vi "CheckIfStartModuleScriptExistsinINIFile.vi"(8 "error in":errorcluster, 11 "OrigTestTreeTags":string[](array[string])) -> (0 "error out":errorcluster, 1 "Found?":bool, 2 "INIs with Start Module script":T1, 3 "OrigTestTreeTags out":string[](array[string]))   [LabVIEW 2018]
uses:
  TestConfiguration.ctl
  <vilib>/Utility/config.llb/NI_LVConfig.lvlib
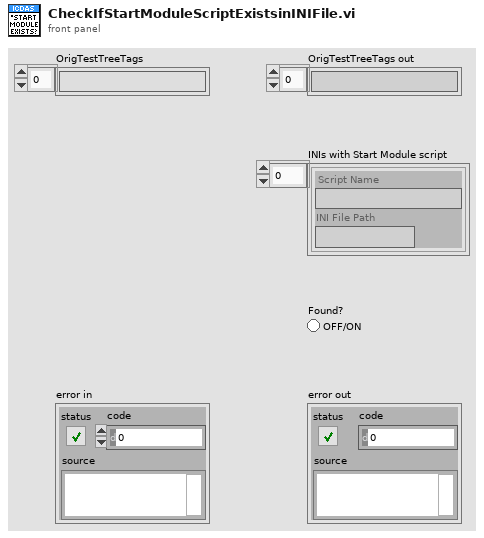
[diagram p1: front panel]
types:
  T1 = typedef "TestConfiguration.ctl" = cluster{"Script Name":string, "INI File Path":string}[]
  T2 = cluster{"Script Name":string, "INI File Path":string}
  T3 = typedef "Plugin Tree Tag.ctl" = cluster{"ItemType":T4, "Name":string, "Path":path, "Script":string[]}
  T4 = typedef "Plugins Tree Item Type.ctl" = enum16{"Plugin", "Instrument", "INI File", "INI Script"}
  T5 = typedef "NI_LVConfig.lvlib/Config Data RefNum.ctl" = refnum<k1>
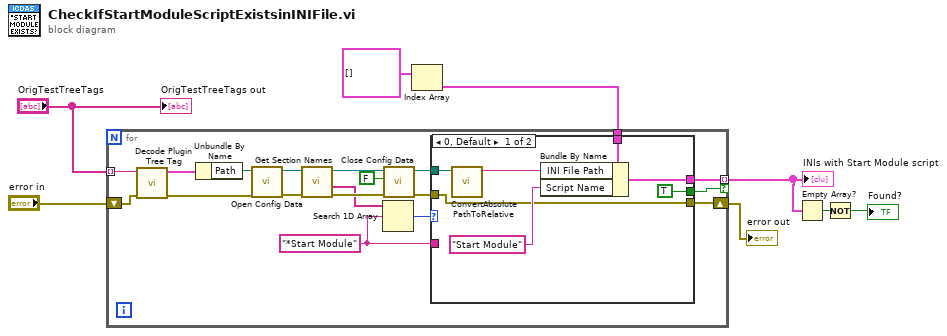
[diagram p0: block diagram]
diagram:
  n1 = Index Array(array=T1 [] ("Test Configuration")) -> (element=w5:T2)  [unwired: 1 in]
  n2 = for {
    tunnel: "OrigTestTreeTags" -> [w27] mode=indexing
    shift-right: [w12] -> w4
    shift-left: "error in" -> [w14]
    tunnel: w5 -> [w11]
    tunnel: [w10] -> w3 mode=indexing if=w9
    w13 = "*Start Module" ("element")
    n3 = call "Decode Plugin Tree Tag.vi"("error in (no error)"=w14, "Tag"=w27) -> ("error out"=w15:errorcluster, "Plugin Tree Tag"=w26:T3)  [unwired: 8 in]
    n4 = Unbundle By Name(w26) -> ("Path"=w19:path)
    n5 = call <vilib>:"Open Config Data.vi"("error in (no error)"=w15, "configuration file path"=w19) -> ("error out"=w22:errorcluster, "refnum"=w21:T5)  [unwired: 7 in, 1 out]
    n6 = call <vilib>:"Get Section Names.vi"("error in (no error)"=w22, "refnum"=w21) -> ("error out"=w24:errorcluster, "section names"=w23:string[], "refnum out"=w25:T5)  [unwired: 7 in]
    n7 = Search 1D Array(1D array=w23, element=w13) -> (index of element=w18:i32)  [unwired: 1 in]
    n8 = call <vilib>:"Close Config Data.vi"("error in (no error)"=w24, "write file if changed (T)"=FALSE, "refnum"=w25) -> ("error out"=w16:errorcluster, "file path"=w17:path)  [unwired: 7 in]
    n9 = case shown="0, Default" w18 {
      tunnel: w17 -> [w34 _]
      tunnel: w16 -> [w30 w36]
      tunnel: w13 -> [_ _]
      tunnel: [w30 w36] -> w12
      tunnel: w11 -> [w33 w35]
      tunnel: [w29 w35] -> w10
      tunnel: [TRUE _] -> w9
      frame 0, Default {
        n10 = call "ConvertAbsolutePathToRelative.vi"("Absolute Path"=w34) -> ("RelativePath"=w32:string)  [unwired: 10 in]
        n11 = Bundle By Name(cluster=w33, "INI File Path"=w32, "Script Name"="Start Module" ("element")) -> (w29:T2)
      }
      frame -1 {
      }
    }
  }
  "INIs with Start Module script" <- w3
  "error out" <- w4
  n12 = Empty Array?(array=w3) -> (empty?=w2:bool)
  n13 = Not(x=w2) -> (.not. x?=→"Found?":bool)
  "OrigTestTreeTags out" <- "OrigTestTreeTags"
